vi "Mouseover.vi"(8 "error in (no error)":errorcluster, 10 "Byte Position":i32, 11 "BreadcrumbNavigation in":refnum<class "BreadcrumbNavigator.lvclass">) -> (0 "error out":errorcluster, 3 "BreadcrumbNavigation out":refnum<class "BreadcrumbNavigator.lvclass">)   [LabVIEW 2015, in "BreadcrumbNavigator.lvclass"]
uses:
  BreadcrumbNavigator.lvclass
  <vilib>/Utility/miscctls.llb/LVSelectionTypeDef.ctl
  BreadcrumbNavigator.lvclass/BreadcrumbNavigator.ctl
  Read Strings[].vi
  Read CurrentLeftMostItem.vi
  Read Delimeter.vi
  <vilib>/Utility/cursorutil.llb/Set Cursor (Icon Pict).vi
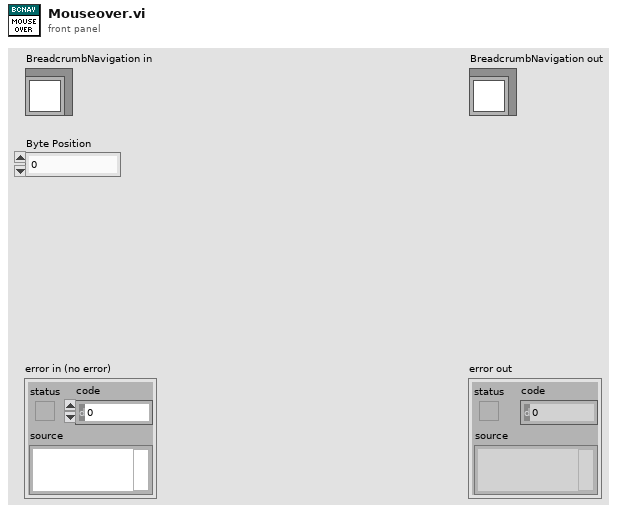
[diagram p1: front panel]
types:
  T1 = typedef "LVSelectionTypeDef.ctl" = cluster{"Selection Start":u32, "Selection End":u32}
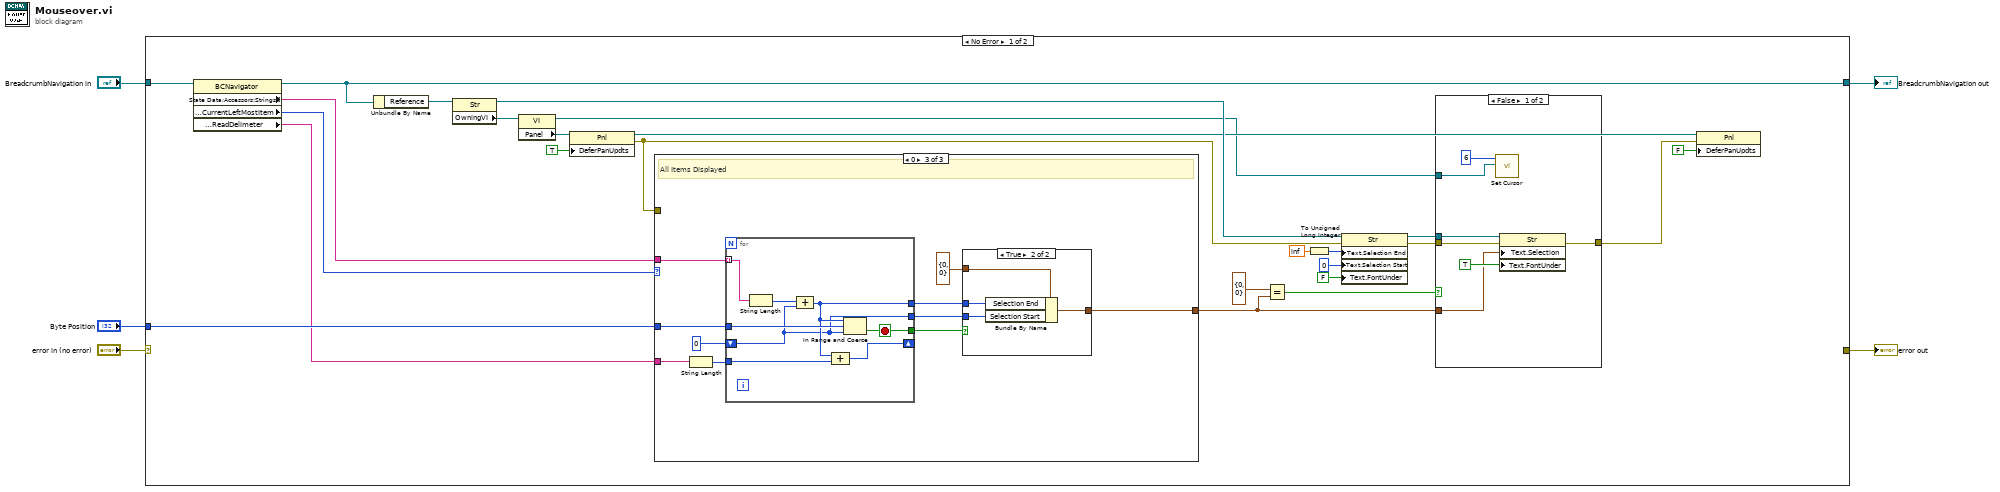
[diagram p0: block diagram]
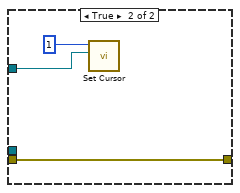
[diagram p2: hidden frame]
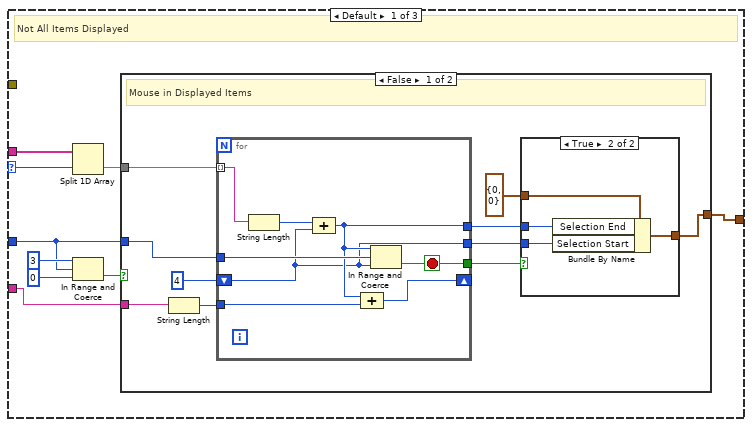
[diagram p3: hidden frame]
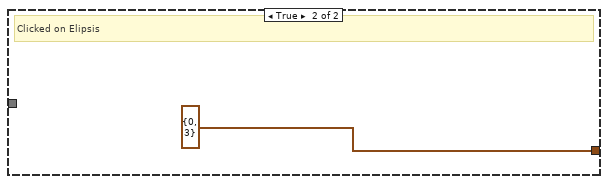
[diagram p5: hidden frame]
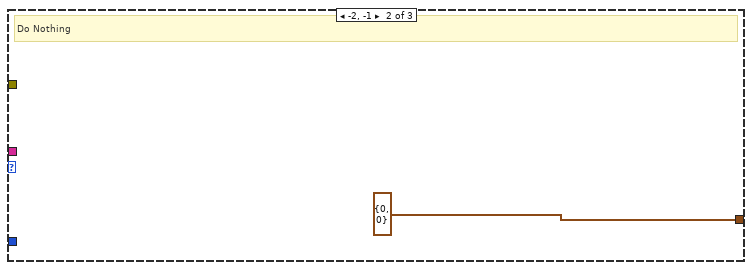
[diagram p6: hidden frame]
diagram:
  n1 = case shown="No Error" "error in (no error)" {
    selector: "error in (no error)" -> [_ w99]
    tunnel: [_ w99] -> w4
    tunnel: [w25 w98] -> w2
    tunnel: "BreadcrumbNavigation in" -> [w30 w98]
    tunnel: "Byte Position" -> [w27 _]
    frame No Error {
      n2 = property class="BCNavigator"(reference=w30) -> (reference out=w25:refnum<class "BreadcrumbNavigator.lvclass">, "State Data:Accessors:Strings[]"=w29:string[], "State Data:Accessors:CurrentLeftMostItem"=w28:i32, "State Data:Accessors:ReadDelimeter"=w26:string)  [unwired: 1 in, 1 out]
      n3 = Unbundle By Name(w25) -> ("Reference"=w24:refnum<vi>)
      n4 = property class="Str"(reference=w24) -> (reference out=w20:refnum<vi>, "OwningVI"=w23:refnum<vi>)  [unwired: 1 in, 1 out]
      n5 = property class="VI"(reference=w23) -> (reference out=w6:refnum<vi>, "Panel"=w22:refnum<vi>)  [unwired: 1 in, 1 out]
      n6 = property class="Pnl"(reference=w22, "DeferPanUpdts"=TRUE ("Defer Panel Updates")) -> (reference out=w15:refnum<vi>, error out=w16:errorcluster)  [unwired: 1 in]
      n7 = case shown="0" w28 {
        selector: w28 -> [w48 _ _]
        tunnel: w29 -> [w49 _ w83]
        tunnel: w27 -> [w43 _ w82]
        tunnel: w26 -> [w42 _ w84]
        tunnel: w16 -> [_ _ _]
        tunnel: [w41 T1 {"Selection Start"=0, "Selection End"=0} ("Text.Selection") w75] -> w19
        frame Default {
          # "Not All Items Displayed"
          n8 = Split 1D Array(array=w49, index=w48) -> (second subarray=w44:string[])  [unwired: 1 out]
          n9 = In Range and Coerce(upper limit=3, x=w43, lower limit=0) -> (In Range?=w45:bool)  [unwired: 1 out]
          n10 = case shown="False" w45 {
            tunnel: w44 -> [w57 _]
            tunnel: w43 -> [w56 _]
            tunnel: w42 -> [w55 _]
            tunnel: [w51 T1 {"Selection Start"=0, "Selection End"=3} ("Text.Selection")] -> w41
            frame False {
              # "Mouse in Displayed Items"
              n11 = String Length(string=w55) -> (length=w59:i32)
              n12 = for {
                tunnel: w57 -> [w69] mode=indexing
                tunnel: w56 -> [w72]
                shift-right: [w70] -> _
                shift-left: 4 -> [w66]
                tunnel: w59 -> [w71]
                tunnel: [w67] -> w53
                tunnel: [w66] -> w52
                tunnel: [w65] -> w50
                stop <- w65 stop-if-true
                n13 = String Length(string=w69) -> (length=w68:i32)
                n14 = Compound Arithmetic op=ADD(w68, w66) -> (w67:i32)
                n15 = Compound Arithmetic op=ADD(w67, w71) -> (w70:i32)
                n16 = In Range and Coerce(upper limit=w67, x=w72, lower limit=w66) -> (In Range?=w65:bool)  [unwired: 1 out]
              }
              n17 = case shown="True" w50 {
                tunnel: T1 {"Selection Start"=0, "Selection End"=0} ("Text.Selection") -> [w60 w64]
                tunnel: w53 -> [_ w63]
                tunnel: w52 -> [_ w62]
                tunnel: [w60 w61] -> w51
                frame False {
                }
                frame True {
                  n18 = Bundle By Name(cluster=w64, "Selection End"=w63, "Selection Start"=w62) -> (w61:T1)
                }
              }
            }
            frame True {
              # "Clicked on Elipsis"
            }
          }
        }
        frame -2, -1 {
          # "Do Nothing"
        }
        frame 0 {
          # "All Items Displayed"
          n19 = String Length(string=w84) -> (length=w80:i32)
          n20 = for {
            tunnel: w83 -> [w94] mode=indexing
            tunnel: w82 -> [w97]
            shift-right: [w95] -> _
            shift-left: 0 -> [w91]
            tunnel: w80 -> [w96]
            tunnel: [w92] -> w78
            tunnel: [w91] -> w77
            tunnel: [w90] -> w76
            stop <- w90 stop-if-true
            n21 = String Length(string=w94) -> (length=w93:i32)
            n22 = Compound Arithmetic op=ADD(w93, w91) -> (w92:i32)
            n23 = Compound Arithmetic op=ADD(w92, w96) -> (w95:i32)
            n24 = In Range and Coerce(upper limit=w92, x=w97, lower limit=w91) -> (In Range?=w90:bool)  [unwired: 1 out]
          }
          n25 = case shown="True" w76 {
            tunnel: T1 {"Selection Start"=0, "Selection End"=0} ("Text.Selection") -> [w85 w89]
            tunnel: w78 -> [_ w88]
            tunnel: w77 -> [_ w87]
            tunnel: [w85 w86] -> w75
            frame False {
            }
            frame True {
              n26 = Bundle By Name(cluster=w89, "Selection End"=w88, "Selection Start"=w87) -> (w86:T1)
            }
          }
        }
      }
      n27 = Equal?(x=T1 {"Selection Start"=0, "Selection End"=0}, y=w19) -> (x = y?=w7:bool)
      n28 = To Unsigned Long Integer(number=inf) -> (unsigned 32bit integer=w11:u32)
      n29 = property class="Str"(reference=w20, error in=w16, "Text.Selection End"=w11, "Text.Selection Start"=u32 0 ("Text.Selection:Start"), "Text.FontUnder"=FALSE ("Text.Font:Underline")) -> (reference out=w10:refnum<vi>, error out=w9:errorcluster)
      n30 = case shown="False" w7 {
        tunnel: w10 -> [w36 _]
        tunnel: w9 -> [w35 w40]
        tunnel: [w34 w40] -> w17
        tunnel: w19 -> [w33 _]
        tunnel: w6 -> [w32 w38]
        frame False {
          n31 = call-poly <vilib>:"Set Cursor.vi"("VI reference (current VI)"=w32, "icon"=u16 6) -> ()  [unwired: 8 in, 2 out]
          n32 = property class="Str"(reference=w36, error in=w35, "Text.Selection"=w33, "Text.FontUnder"=TRUE ("Text.Font:Underline")) -> (error out=w34:errorcluster)  [unwired: 1 out]
        }
        frame True {
          n33 = call-poly <vilib>:"Set Cursor.vi"("VI reference (current VI)"=w38, "icon"=u16 1) -> ()  [unwired: 8 in, 2 out]
        }
      }
      n34 = property class="Pnl"(reference=w15, error in=w17, "DeferPanUpdts"=FALSE ("Defer Panel Updates")) -> ()  [unwired: 2 out]
    }
    frame Error {
    }
  }
  "error out" <- w4
  "BreadcrumbNavigation out" <- w2
